vi "Read EDR.vi"(11 "Main UI in":refnum<class "Main UI.lvclass">) -> (2 "EDR":refnum<vi>, 3 "Main UI out":refnum<class "Main UI.lvclass">)   [LabVIEW 2011, in "Main UI.lvclass"]
uses:
  Main UI.lvclass
  Main UI.lvclass/Main UI.ctl
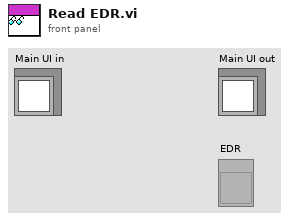
[diagram p1: front panel]
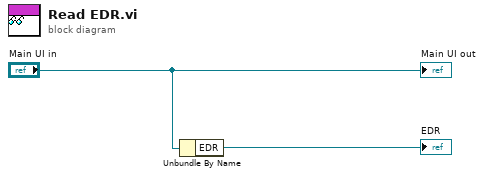
[diagram p0: block diagram]
diagram:
  n1 = Unbundle By Name("Main UI in") -> ("EDR"=→"EDR":refnum<vi>)
  "Main UI out" <- "Main UI in"
